vi "From Serial Form.vi"(6 "Serial Version":T1, 10 "Deserializer in":refnum<class "Deserializer.lvclass">, 11 "Instrument in":refnum<class "Instrument.lvclass">) -> (0 "error out":errorcluster, 2 "Deserializer out":refnum<class "Deserializer.lvclass">, 3 "Instrument out":refnum<class "Instrument.lvclass">)   [LabVIEW 2012]
uses:
  <userlib>/Serialization/Serializable/Serializable.lvclass
  <userlib>/Serialization/Serializable/Remove String.vi
  <userlib>/Serialization/Serialization Common/Serial Version.ctl
  <userlib>/Serialization/Serialization Common/Serialization Common.lvlib
  <userlib>/Serialization/Deserializer/Deserializer.lvclass
  Instrument.lvclass
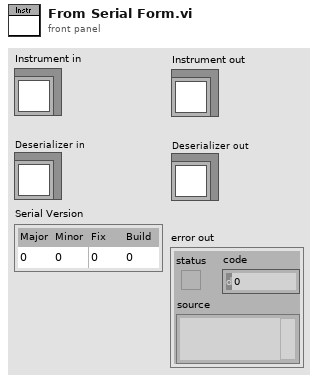
[diagram p1: front panel]
types:
  T1 = typedef "Serialization Common.lvlib/Serial Version.ctl" = cluster{"Major":u16, "Minor":u16, "Fix":u16, "Build":u16}
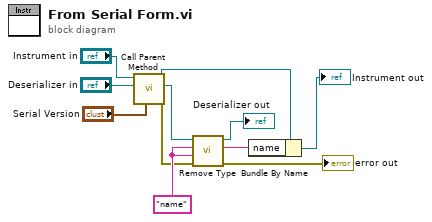
[diagram p0: block diagram]
diagram:
  w8 = "name" ("Name")
  n1 = call-parent "Call Parent Method"("Serial Version"="Serial Version", "Deserializer in"="Deserializer in", "Serializable in"="Instrument in") -> ("error out"=w5:errorcluster, "Deserializer out"=w7:refnum<class "Deserializer.lvclass">, "Serializable out"=w3:refnum<class "Serializable.lvclass">)  [unwired: 6 in]
  n2 = call-poly <userlib>:"Remove Type.vi"("error in (no error)"=w5, "Name"=w8, "Default Value"=w8, "Deserializer in"=w7) -> ("error out"=→"error out":errorcluster, "String"=w2:string, "Deserializer out"=→"Deserializer out":refnum<class "Deserializer.lvclass">)  [unwired: 4 in, 1 out]
  n3 = Bundle By Name(cluster=w3, "name"=w2) -> (→"Instrument out":refnum<class "Serializable.lvclass">)
